vi "Real Wind Monitor USB.vi"() -> ()   [LabVIEW 2026]
uses:
  Real Wind Sample.ctl
  <vilib>/Instr/_visa.llb/VISA Configure Serial Port (Instr).vi
panel:
  out "Serial Errors":errorcluster
  out "Raw Master Packet":string
  out "Connection Good?":bool
  in  "VISA resource name":refnum<visa-resource-name>
  in  "Direction Modbus Response":string
  out "Error Logs:":errorcluster
  out "CSV Row Preview":string
  in  "CSV File Path":path
  in  "Enable Logging?\nDown=OFF btw":bool
  out "Wind Speed History":dbl(graph)
  out "Wind Direction History":dbl(graph)
  out "Is The Coming Packet Valid?":bool
  out "Current Wind Sample:":T1
  in  "Speed Modbus Response":string
  in  "?":bool
  # "These down two are for tests incase\nyou dont have real data flowing (hexa):\n---------------------------------------------"
  # "Stop All"
  # "-----------------------------------------------"
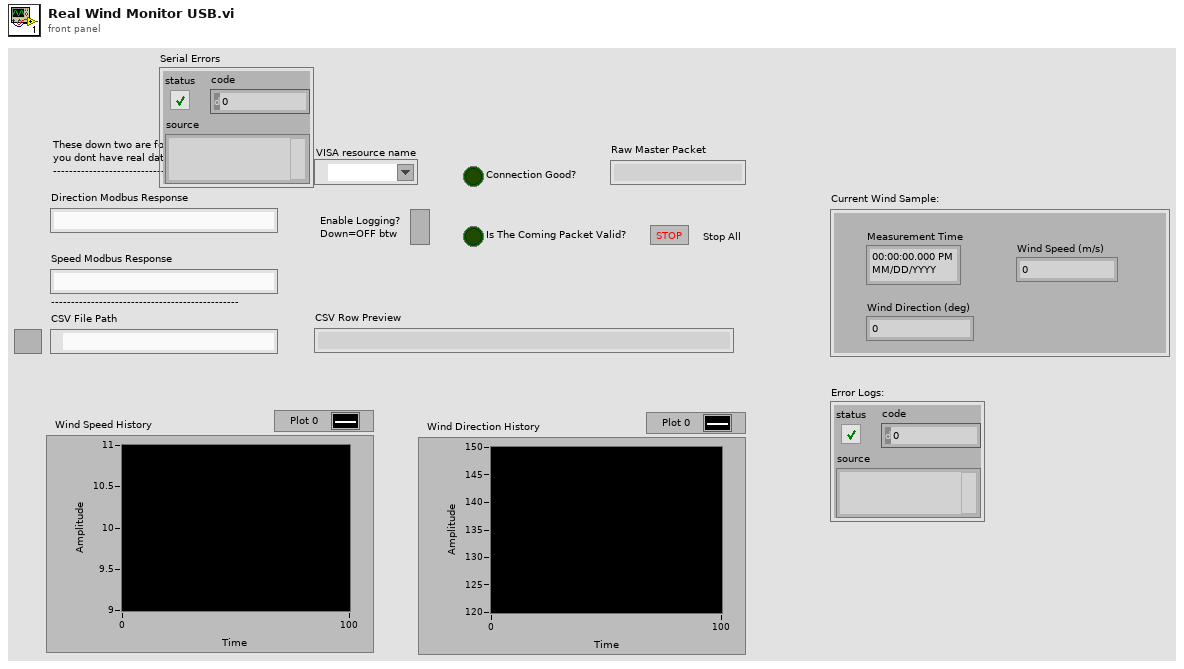
[diagram p1: front panel]
types:
  T1 = typedef "Real Wind Sample.ctl" = cluster{"Measurement Time":timestamp, "Wind Direction (deg)":dbl, "Wind Speed (m/s)":dbl}
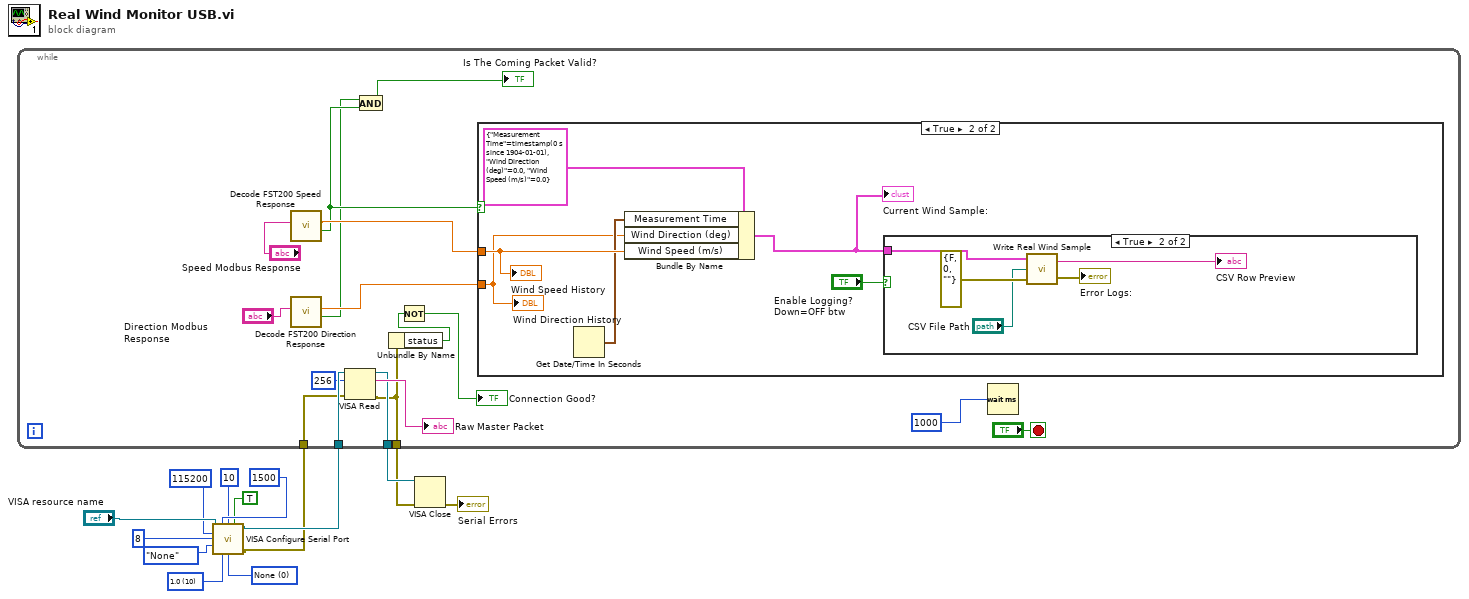
[diagram p0: block diagram]
diagram:
  w6 = u16 0 items=["None", "XON/XOFF", "RTS/CTS", "XON/XOFF & RTS/CTS", "DTR/DSR", "XON/XOFF & DTR/DSR"] ("flow control (0:none)")
  w7 = u16 10 items=["1.0"=10, "1.5"=15, "2.0"=20] ("stop bits (10: 1 bit)")
  n1 = call-poly "VISA Configure Serial Port"("VISA resource name"="VISA resource name", "timeout (10sec)"=u32 1500, "termination char\n(0xA = '\\n' = LF)"=u8 10 ("termination char\n(0xA = '\\n' = LF)"), "Enable Termination\nChar (T)"=TRUE ("Enable Termination\nChar (T)"), "baud rate (9600)"=u32 115200, "data bits (8)"=u16 8, "parity (0:none)"=enum16{"None", "Odd", "Even", "Mark", "Space"}."None", "stop bits (10: 1 bit)"=w7, "flow control (0:none)"=w6) -> ("VISA resource name out"=w5:refnum<visa-resource-name>, "error out"=w4:errorcluster)  [unwired: 5 in]
  n2 = while {
    tunnel: w5 -> [w22]
    tunnel: w4 -> [w21]
    tunnel: [w18] -> w3
    tunnel: [w17] -> w2
    stop <- "?" stop-if-true
    n3 = call "Decode FST200 Speed Response.vi"("Modbus Response"="Speed Modbus Response") -> ("Frame Valid?"=w25:bool, "Wind Speed (m/s)"=w28:dbl)  [unwired: 9 in]
    n4 = call "Decode FST200 Direction Response.vi"("Direction Modbus Response"="Direction Modbus Response") -> ("Frame Valid?"=w24:bool, "Wind Direction (deg)"=w27:dbl)  [unwired: 9 in]
    n5 = VISA Read(VISA resource name=w22, byte count=u32 256, error in (no error)=w21) -> (VISA resource name out=w18:refnum<visa-resource-name>, read buffer=→"Raw Master Packet":string, error out=w17:errorcluster)  [unwired: 1 out]
    n6 = And(x=w24, y=w25) -> (x .and. y?=→"Is The Coming Packet Valid?":bool)
    n7 = Unbundle By Name(w17) -> ("status"=w16:bool)
    n8 = Not(x=w16) -> (.not. x?=→"Connection Good?":bool)
    n9 = case shown="True" w25 {
      tunnel: w28 -> [_ w36]
      tunnel: w27 -> [_ w32]
      frame False {
      }
      frame True {
        n10 = Get Date/Time In Seconds() -> (seconds since 1Jan1904=w35:timestamp)
        n11 = Bundle By Name(cluster=T1 {"Measurement Time"=timestamp(0 s since 1904-01-01), "Wind Direction (deg)"=0.0, "Wind Speed (m/s)"=0.0} ("Real Wind Sample"), "Measurement Time"=w35, "Wind Direction (deg)"=w32, "Wind Speed (m/s)"=w36) -> (w33:T1)
        "Current Wind Sample:" <- w33
        n12 = case shown="True" "Enable Logging?\nDown=OFF btw" {
          tunnel: w33 -> [_ w39]
          frame False {
          }
          frame True {
            n13 = call "Write Real Wind Sample.vi"("error in"=errorcluster {"status"=FALSE, "code"=0, "source"=""}, "CSV File Path"="CSV File Path", "Real Wind Sample"=w39) -> ("error out"=→"Error Logs:":errorcluster, "CSV Row Preview"=→"CSV Row Preview":string)
          }
        }
        "Wind Direction History" <- w32
        "Wind Speed History" <- w36
      }
    }
    n14 = Wait (ms)(milliseconds to wait=u32 1000) -> ()  [unwired: 1 out]
  }
  n15 = VISA Close(VISA resource name=w3, error in (no error)=w2) -> (error out=→"Serial Errors":errorcluster)
